vi "Disconnect Site Relays.vi"(0 "TSM context":T1, 11 "error in":errorcluster) -> (4 "TSM context out":T1, 15 "error out":errorcluster)   [LabVIEW 2019]
uses:
  <vilib>/NI_TestStand_SemiconductorModule/NI_TestStand_Semiconductor_Module.lvlibp/PinMap/General/SemiconductorModuleContext.ctl
  <instrlib>/niSwitch/niSwitch.llb/niSwitch Relay Action.ctl
  SSC/SSC Relay Control.vi
  SSC/SSC Relay Control/SSC Relay Control Single Action.vi
  SSC/SSC Relay Control Core.vi
  SSC/Single SSC Relay NI-Switch Control.vi
  SSC/Single SSC Relay Fill Additional Error info.vi
  SSC/SSC Relay Expand Action Array to All Sessions.vi
  TSM/TSM Relay Get Sessions/TSM Relay Pins to Sessions.vi
  <vilib>/Utility/error.llb/Error Cluster From Error Code.vi
  <instrlib>/niSwitch/niSwitch.llb/niSwitch Get Relay Position.vi
  <instrlib>/niSwitch/niSwitch.llb/niSwitch Relay Control.vi
  <vilib>/Utility/High Resolution Polling Wait.vi
  <vilib>/NI_TestStand_SemiconductorModule/NI_TestStand_Semiconductor_Module.lvlibp
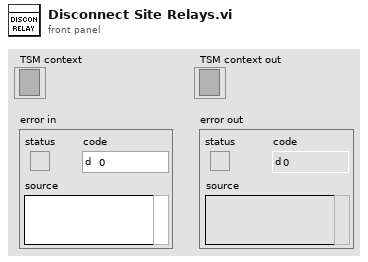
[diagram p1: front panel]
types:
  T1 = typedef "NI_TestStand_Semiconductor_Module.lvlibp/SemiconductorModuleContext.ctl" = refnum<k7>
  T2 = typedef "niSwitch Relay Action.ctl" = i32
  T3 = typedef "TSM SSC Relay.ctl" = cluster{"TSM context":T1, "Pin Query Context":refnum<class "MultiplePinMultipleSessionQueryContext.lvclass">, "TSM Site Numbers":i32[], "SSC Relay":T4[], "Unfiltered Pins":string[], "Filtered Pins":string[], "Filtered Pins Info":T5}
  T4 = typedef "SSC Relay.ctl" = cluster{"Relay":string, "Site":i32, "Session":refnum<k15>, "Channel":string}
  T5 = typedef "TSM Filtered Pins Info.ctl" = cluster{"Unfiltered Pins Count":i32, "Locations":i32[], "Lengths":i32[]}
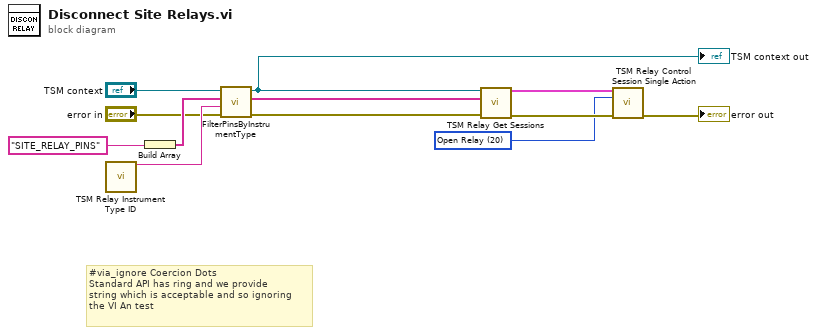
[diagram p0: block diagram]
diagram:
  w7 = T2 20 items=["Open Relay"=20, "Close Relay"=21] ("Relay Action")
  # "#via_ignore Coercion Dots\nStandard API has ring and we provide\nstring which is acceptable and so ignoring\nthe VI An test"
  n1 = call "TSM Relay Instrument Type ID.vi"() -> ("Instrument Type ID"=w10:string)  [unwired: 15 in]
  n2 = Build Array("SITE_RELAY_PINS" ("String")) -> (w11:string[])
  n3 = call <vilib>:"FilterPinsByInstrumentType.vi"("error in (no error)"="error in", "Instrument Type Id"=w10, "Pins"=w11, "Semiconductor Module Context"="TSM context") -> ("error out"=w9:errorcluster, "Filtered Pins"=w5:tag[], "Semiconductor Module Context Out"=w6:T1)  [unwired: 5 in]
  "TSM context out" <- w6
  n4 = call-poly "TSM Relay Get Sessions.vi"("TSM context"=w6, "Relay Pins"=w5, "error in"=w9) -> ("TSM Relay"=w1:T3, "error out"=w8:errorcluster)  [unwired: 11 in]
  n5 = call "TSM Relay Control Session Single Action.vi"("TSM Relay in"=w1, "Relay Action"=w7, "error in"=w8) -> ("error out"=→"error out":errorcluster)  [unwired: 10 in, 2 out]
